vi "TCPcloseConnection.vi"(0 "DashboardServer in":refnum<class "Dashboard Server.lvclass">, 5 "error in (no error)":errorcluster) -> (14 "DashboardServer out":refnum<class "Dashboard Server.lvclass">, 19 "error out":errorcluster)   [LabVIEW 2019, in "Dashboard Server.lvclass"]
uses:
  Dashboard Server.lvclass
  Dashboard Server.lvclass/Dashboard Server.ctl
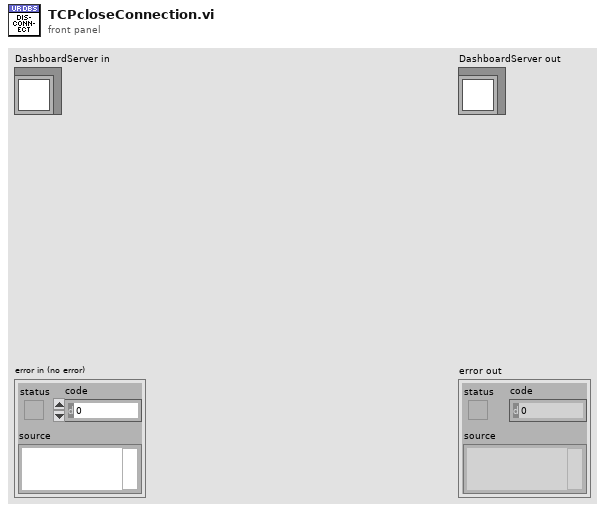
[diagram p1: front panel]
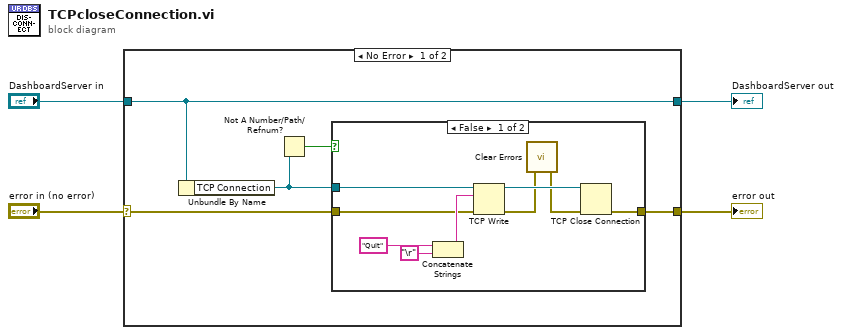
[diagram p0: block diagram]
diagram:
  n1 = case shown="No Error" "error in (no error)" {
    selector: "error in (no error)" -> [w7 w21]
    tunnel: [w9 w21] -> w3
    tunnel: [w8 w20] -> w1
    tunnel: "DashboardServer in" -> [w8 w20]
    frame No Error {
      n2 = Unbundle By Name(w8) -> ("TCP Connection"=w6:refnum<k5>)
      n3 = Not A Number/Path/Refnum?(number/path/refnum=w6) -> (NaN/Path/Refnum?=w5:bool)
      n4 = case shown="False" w5 {
        tunnel: [w18 w19] -> w9
        tunnel: w7 -> [w14 w19]
        tunnel: w6 -> [w10 _]
        frame False {
          n5 = Concatenate Strings("Quit" ("string"), "\r") -> (w16:string)
          n6 = TCP Write(connection ID=w10, data in=w16, error in (no error)=w14) -> (connection ID out=w15:refnum<k5>, error out=w12:errorcluster)  [unwired: 1 in, 1 out]
          n7 = call <vilib>:"Clear Errors.vi"("error in (no error)"=w12) -> ("error out"=w11:errorcluster)  [unwired: 5 in, 1 out]
          n8 = TCP Close Connection(connection ID=w15, error in (no error)=w11) -> (error out=w18:errorcluster)  [unwired: 1 in, 1 out]
        }
        frame True {
        }
      }
    }
    frame Error {
    }
  }
  "error out" <- w3
  "DashboardServer out" <- w1
